vi "Get Resource Type.vi"(11 "SPI in":refnum<class "SPI.lvclass">) -> (2 "Resource Type":string)   [LabVIEW 2020, in "CTI.lvlib" / "SPI.lvclass"]
uses:
  SPI.lvclass
  SPI.lvclass/SPI.ctl
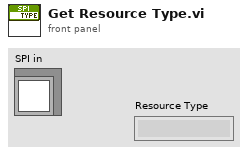
[diagram p1: front panel]
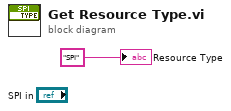
[diagram p0: block diagram]
diagram:
  "Resource Type" <- "SPI" ("Resource Type")
